vi "wait for udp trigger.vi"(8 "error in (no error)":errorcluster) -> (0 "No error":errorcluster)   [LabVIEW 2020]
uses:
  DeviceController/DeviceGlobals.vi
  <vilib>/Utility/tcp.llb/UDP Multicast Read-Only Open.vi
panel:
  out "ms timestamp network trigger":dbl
  out "x-y":dbl
  out "1st read":errorcluster
  out "2nd udp error":errorcluster
  out "data out 2":string
  out "data out":string
  out "loops to clear buffer":i32
  out "NetTrigger Time Stamp":timestamp
  out "current time":timestamp
  out "wait time":u32
  out "connection ID":refnum<k16>
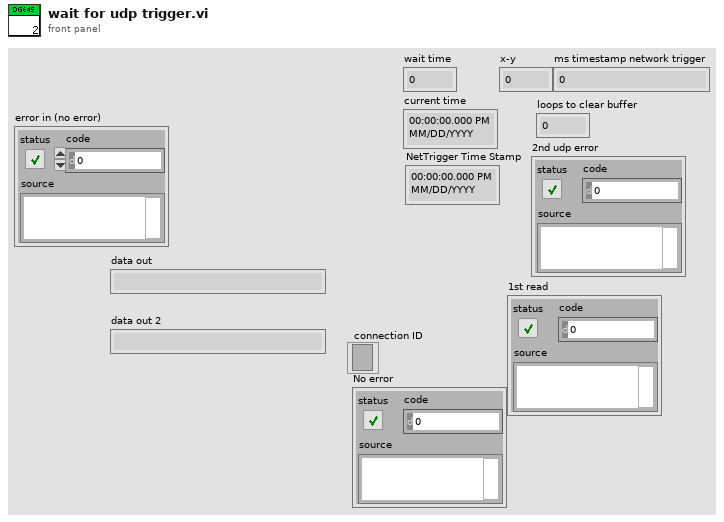
[diagram p1: front panel]
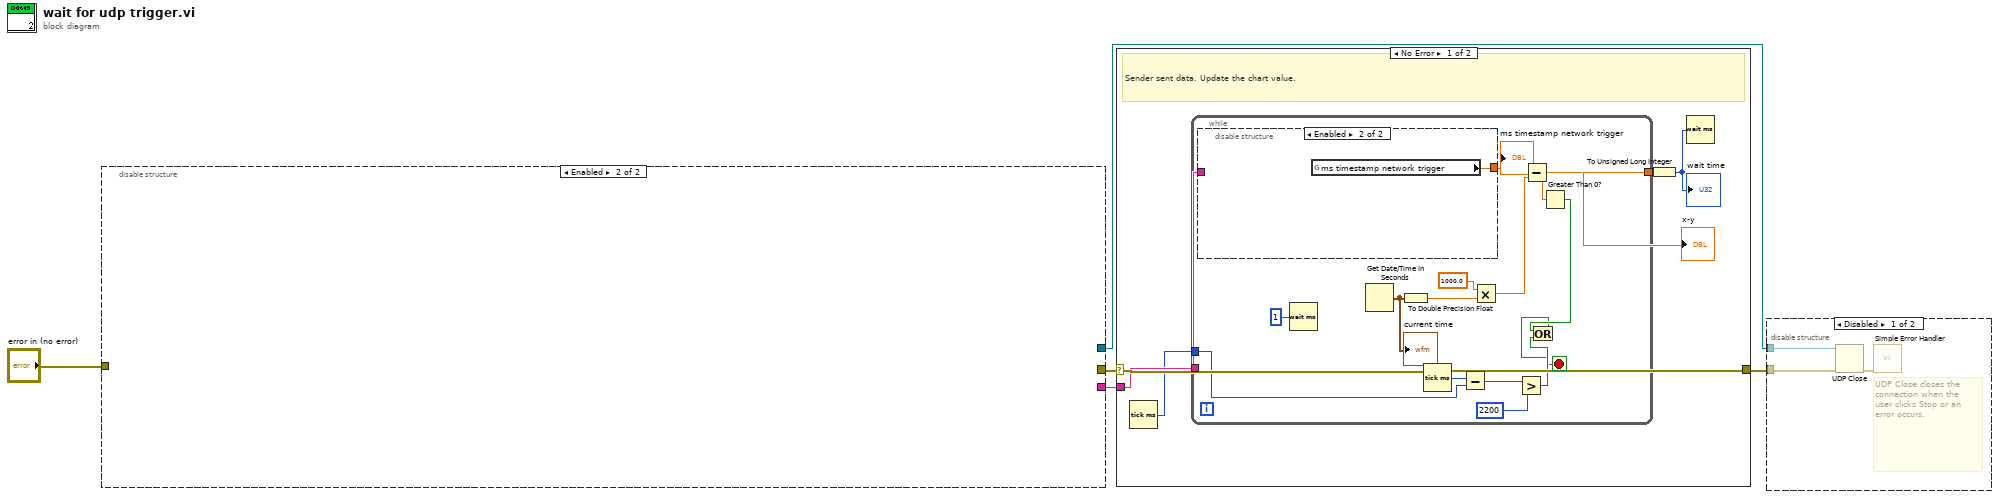
[diagram p0: block diagram]
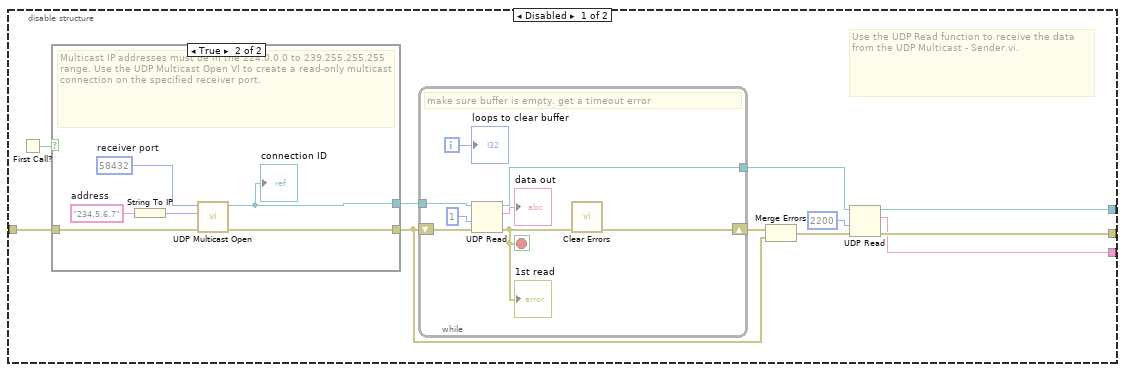
[diagram p2: hidden frame]
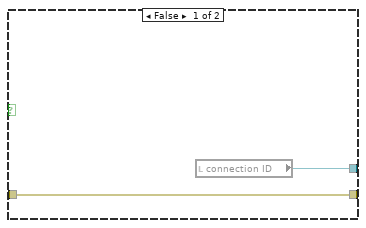
[diagram p3: hidden frame]
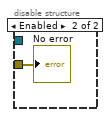
[diagram p4: hidden frame]
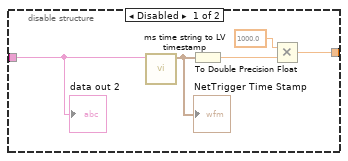
[diagram p5: hidden frame]
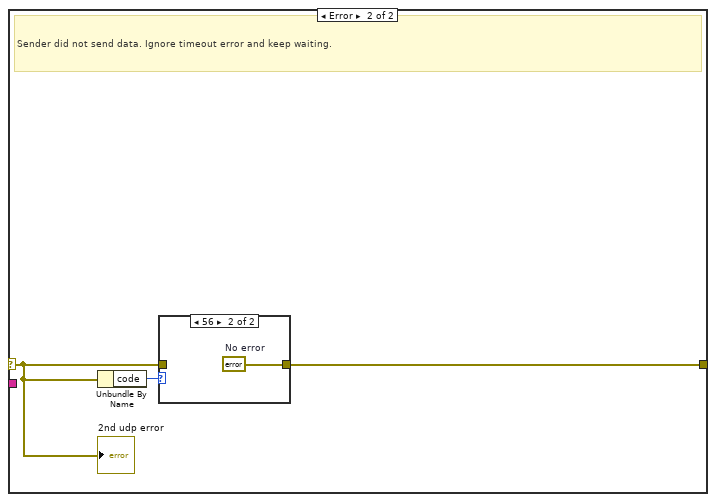
[diagram p6: hidden frame]
diagram:
  n1 = disable-structure shown="Enabled" {
    disable-tunnel: "error in (no error)" -> [w16 _]
    disable-tunnel: [w14 _] -> w4
    disable-tunnel: [w13 _] -> w3
    disable-tunnel: [w11 _] -> w1
    frame Disabled {
      # "Use the UDP Read function to receive the data from the UDP Multicast - Sender.vi."
      n2 = First Call?() -> (First Call?: T/F=w15:bool)
      n3 = case shown="True" w15 {
        tunnel: [w26 w31] -> w9
        tunnel: [w25 w27] -> w7
        tunnel: w16 -> [w26 w28]
        frame False {
          n4 = local read "connection ID"() -> (w25:refnum<k16>)
        }
        frame True {
          w30 = u16 58432  # receiver port
          w32 = "234.5.6.7"  # address
          # "Multicast IP addresses must be in the 224.0.0.0 to 239.255.255.255 range. Use the UDP Multicast Open VI to create a read-only multicast connection on the specified receiver port."
          n5 = String To IP(1:w32) -> (0:w29:u32)
          n6 = call-poly <vilib>:"UDP Multicast Open.vi"("error in (no error)"=w28, "multicast addr"=w29, "port"=w30) -> ("error out"=w31:errorcluster, "connection ID"=w27:refnum<k16>)  [unwired: 6 in, 1 out]
          "connection ID" <- w27
        }
      }
      n7 = while {
        shift-right: [w23] -> w10
        shift-left: w9 -> [w22]
        tunnel: w7 -> [w20]
        tunnel: [w19] -> w6
        i -> [w18]
        stop <- w21 stop-if-true
        # "make sure buffer is empty. get a timeout error"
        n8 = UDP Read(connection ID=w20, timeout ms (25000)=1, 8:w22) -> (data out=→"data out":string, error out=w21:errorcluster, 3:w19:refnum<k16>)  [unwired: 3 out]
        "1st read" <- w21
        n9 = call <vilib>:"Clear Errors.vi"("error in (no error)"=w21) -> ("error out"=w23:errorcluster)  [unwired: 5 in, 1 out]
        "loops to clear buffer" <- w18
      }
      n10 = Merge Errors(w10, w9) -> (w8:errorcluster)
      n11 = UDP Read(connection ID=w6, timeout ms (25000)=2200, 8:w8) -> (data out=w13:string, error out=w14:errorcluster, 3:w11:refnum<k16>)  [unwired: 3 out]
    }
    frame Enabled {
    }
  }
  n12 = case shown="No Error" w4 {
    selector: w4 -> [w37 w60]
    tunnel: w3 -> [w36 _]
    tunnel: [w37 w59] -> w2
    frame No Error {
      # "Sender sent data. Update the chart value."
      n13 = Tick Count (ms)() -> (millisecond timer value=w33:u32)
      n14 = while {
        tunnel: w36 -> [w52]
        tunnel: [w46] -> w35
        tunnel: w33 -> [w44]
        stop <- w39 stop-if-true
        n15 = disable-structure shown="Enabled" {
          disable-tunnel: w52 -> [w57 _]
          disable-tunnel: [w53 w58] -> w48
          frame Disabled {
            n16 = call "ms time string to LV timestamp.vi"("String"=w57) -> ("Time Stamp"=w54:timestamp)  [unwired: 10 in]
            "NetTrigger Time Stamp" <- w54
            n17 = To Double Precision Float(number=w54) -> (double precision float=w56:dbl)
            n18 = Multiply(x=1000.0 ("y"), y=w56) -> (x*y=w53:dbl)
            "data out 2" <- w57
          }
          frame Enabled {
            n19 = global read "DeviceGlobals.vi" "ms timestamp network trigger"() -> (w58:dbl)
          }
        }
        "ms timestamp network trigger" <- w48
        n20 = Wait (ms)(milliseconds to wait=u32 1) -> ()  [unwired: 1 out]
        n21 = Get Date/Time In Seconds() -> (seconds since 1Jan1904=w51:timestamp)
        "current time" <- w51
        n22 = To Double Precision Float(number=w51) -> (double precision float=w49:dbl)
        n23 = Tick Count (ms)() -> (millisecond timer value=w45:u32)
        n24 = Subtract(x=w45, y=w44) -> (x-y=w42:u32)
        n25 = Multiply(x=1000.0 ("y"), y=w49) -> (x*y=w47:dbl)
        n26 = Greater?(x=w42, y=u32 2200) -> (0:w40:bool)
        n27 = Subtract(x=w48, y=w47) -> (x-y=w46:dbl)
        n28 = Greater Than 0?(x=w46) -> (x > 0?=w43:bool)
        n29 = Or(x=w43, y=w40) -> (x .or. y?=w39:bool)
      }
      "x-y" <- w35
      n30 = To Unsigned Long Integer(number=w35) -> (unsigned 32bit integer=w34:u32)
      "wait time" <- w34
      n31 = Wait (ms)(milliseconds to wait=w34) -> ()  [unwired: 1 out]
    }
    frame Error {
      # "Sender did not send data. Ignore timeout error and keep waiting."
      n32 = Unbundle By Name(w60) -> ("code"=w61:i32)
      n33 = case shown="56" w61 {
        tunnel: w60 -> [w62 _]
        tunnel: [w62 w63] -> w59
        frame Default {
        }
        frame 56 {
          w63 = errorcluster {"status"=FALSE, "code"=0, "source"=""}  # No error
        }
      }
      "2nd udp error" <- w60
    }
  }
  n34 = disable-structure shown="Disabled" {
    disable-tunnel: w1 -> [w66 _]
    disable-tunnel: w2 -> [w64 w67]
    frame Disabled {
      # "UDP Close closes the connection when the user clicks Stop or an error occurs."
      n35 = UDP Close(connection ID=w66, 8:w64) -> (error out=w65:errorcluster)  [unwired: 1 out]
      n36 = call <vilib>:"Simple Error Handler.vi"("error in (no error)"=w65) -> ()  [unwired: 1 in, 8 out]
    }
    frame Enabled {
      "No error" <- w67
    }
  }
